vi "Process.vi"(8 "error in":errorcluster) -> (0 "error out":errorcluster)   [LabVIEW 2021, in "dcvmDPI_AD7606B_serverImpl.lvlib"]
uses:
  dcvmDPI_AD7606B_serverImpl.lvlib
  controls/configuration.ctl
  controls/session.ctl
  dcvmDPI_AD7606B_server/RPC Messages/dcvmDPI_IdResponse.ctl
  dcvmDPI_AD7606B_server/RPC Messages/dcvmDPI_ErrorResponse.ctl
  dcvmMessageQueue/controls/Message Data.ctl
  dcvmDPI_AD7606B_server/RPC Messages/dcvmDPI_MeasurementRequest.ctl
  dcvmDPI_AD7606B_server/RPC Messages/dcvmDPI_MeasurementResponse.ctl
  dcvmDPI_AD7606B_server/RPC Messages/dcvmDPI_InitializeRequest.ctl
  dcvmDPI_AD7606B_server/RPC Messages/dcvmDPI_InitializeResponse.ctl
  <instrlib>/niDigital/niDigital.llb/niDigital Trigger Digital Edge - Edge.ctl
  dcvmDPI_AD7606B_server/RPC Messages/dcvmDPI_ConfigureRequest.ctl
  dcvmDPI_AD7606B_server/RPC Messages/dcvmDPI_ConfigureResponse.ctl
  dcvmDPI_AD7606B_server/RPC Messages/dcvmDPI_InitiateResponse.ctl
  dcvmDPI_AD7606B_server/RPC Messages/dcvmDPI_CloseResponse.ctl
  dcvmMessageQueue/dcvmMessageQueue.lvlib
  dcvmDPI_AD7606B_server/dcvmDPI_AD7606B_server.lvlib
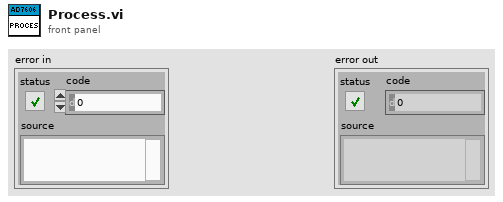
[diagram p1: front panel]
types:
  T1 = typedef "dcvmDPI_AD7606B_serverImpl.lvlib/session.ctl" = cluster{"DPI session":refnum<k15>, "DPI bitfile reference":refnum<k20>}
  T2 = typedef "dcvmDPI_AD7606B_serverImpl.lvlib/configuration.ctl" = cluster{"Input channel":i32, "Sample rate":dbl, "Number of samples":u32, "Measurement Name":string, "reg 0":i32, "reg 1":i32, "Delay ?":bool}
  T3 = typedef "dcvmMessageQueue.lvlib/Message Queues.ctl" = cluster{"gRPC engine":refnum<queue>, "Digital engine":refnum<queue>}
  T4 = typedef "dcvmMessageQueue.lvlib/Message Data.ctl" = cluster{"Action":string, "Value":variant}
  T5 = typedef "dcvmDPI_AD7606B_server.lvlib/dcvmDPI_IdResponse.ctl" = cluster{"name":string, "error":T6}
  T6 = typedef "dcvmDPI_AD7606B_server.lvlib/dcvmDPI_ErrorResponse.ctl" = cluster{"error_number":i32, "error_description":string}
  T7 = typedef "dcvmDPI_AD7606B_server.lvlib/dcvmDPI_MeasurementResponse.ctl" = cluster{"error":T6}
  T8 = typedef "dcvmDPI_AD7606B_server.lvlib/dcvmDPI_MeasurementRequest.ctl" = cluster{"measurement":string}
  T9 = typedef "dcvmDPI_AD7606B_server.lvlib/dcvmDPI_InitializeResponse.ctl" = cluster{"error":T6}
  T10 = typedef "dcvmDPI_AD7606B_server.lvlib/dcvmDPI_InitializeRequest.ctl" = cluster{"device_name":string}
  T11 = typedef "dcvmDPI_AD7606B_server.lvlib/dcvmDPI_ConfigureResponse.ctl" = cluster{"error":T6}
  T12 = enum16{"Initialize", "Write", "Read", "GetBacklog", "Reset"}
  T13 = typedef "dcvmDPI_AD7606B_server.lvlib/dcvmDPI_ConfigureRequest.ctl" = cluster{"digital_capture_samples":u32, "digital_capture_sample_rate":dbl, "input_channel":i32}
  T14 = typedef "dcvmDPI_AD7606B_server.lvlib/dcvmDPI_InitiateResponse.ctl" = cluster{"error":T6}
  T15 = typedef "dcvmDPI_AD7606B_server.lvlib/dcvmDPI_CloseResponse.ctl" = cluster{"error":T6}
  T16 = typedef "niDigital Trigger Digital Edge - Edge.ctl" = i32
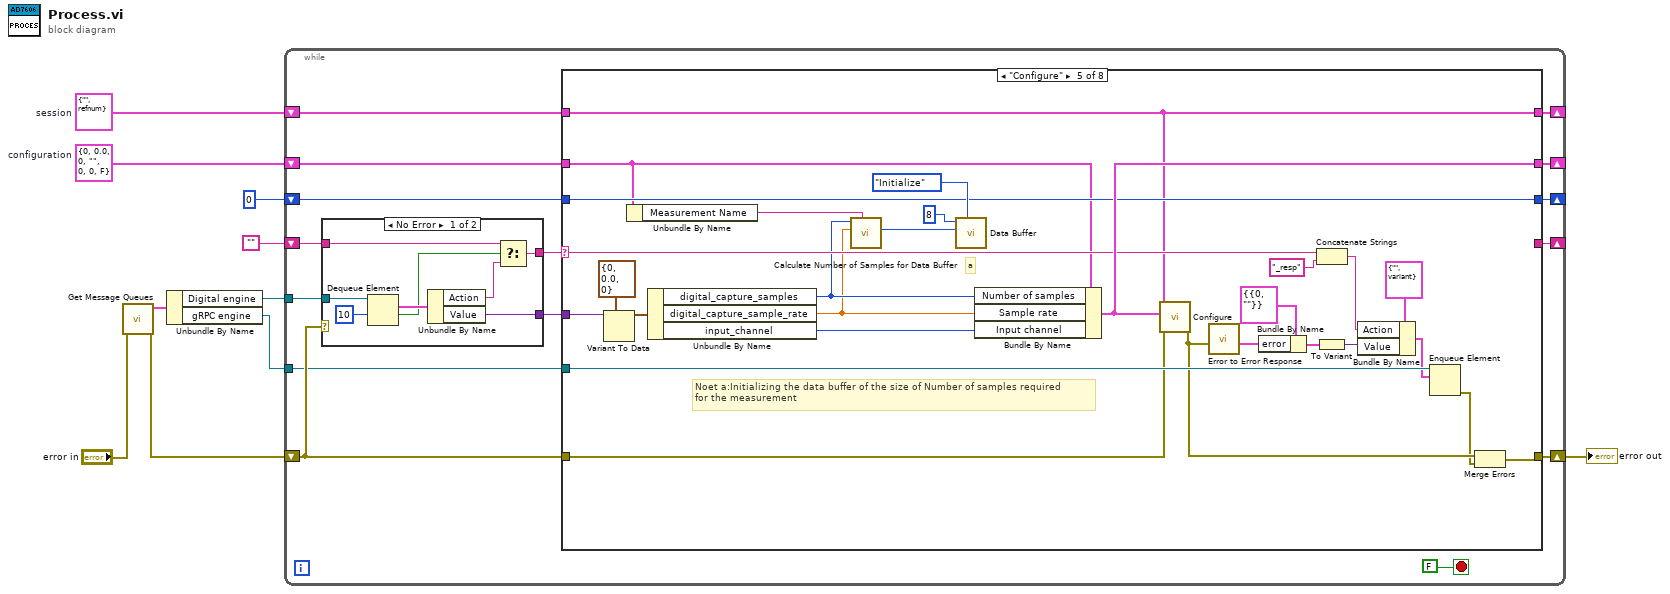
[diagram p0: block diagram]
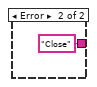
[diagram p2: hidden frame]
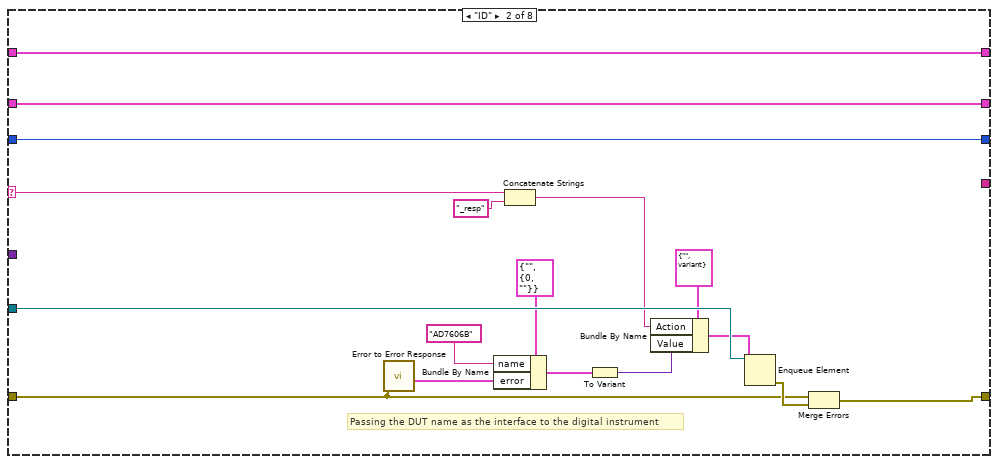
[diagram p4: hidden frame]
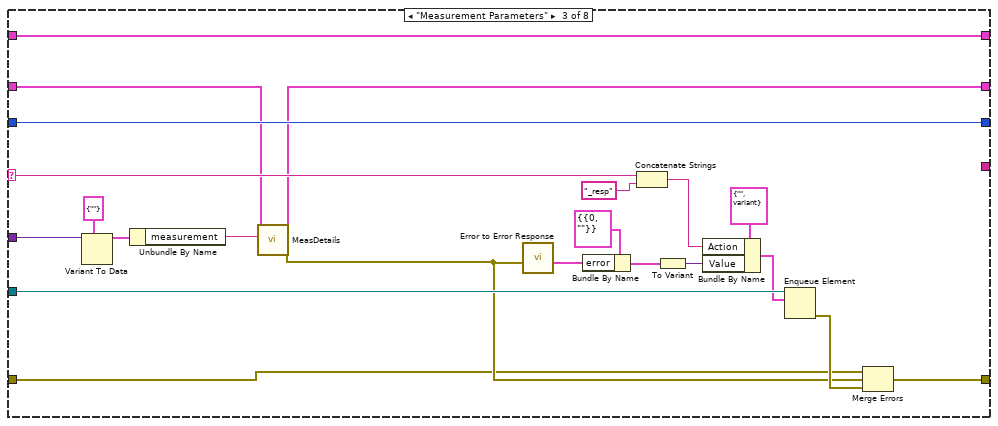
[diagram p5: hidden frame]
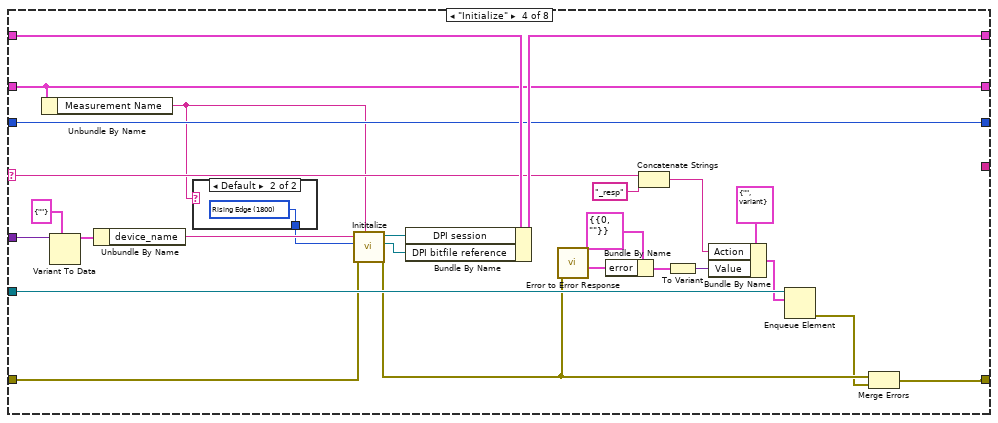
[diagram p6: hidden frame]
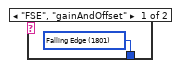
[diagram p7: hidden frame]
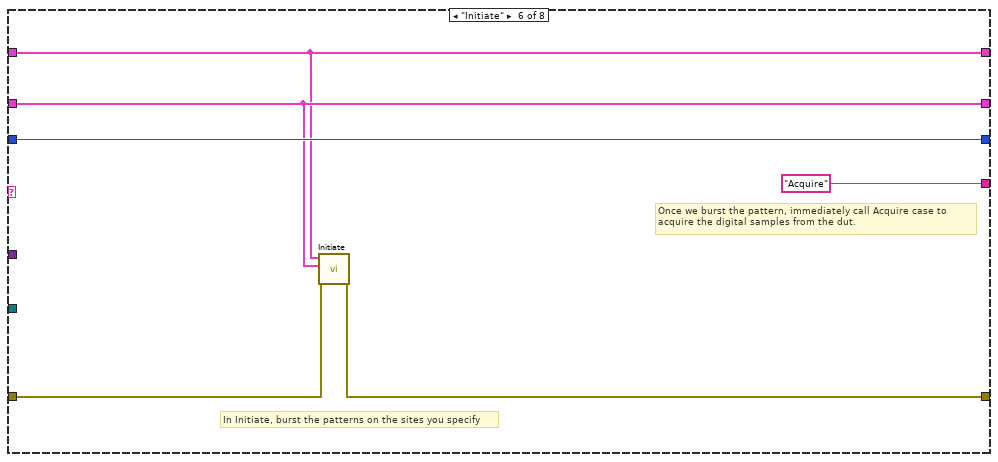
[diagram p8: hidden frame]
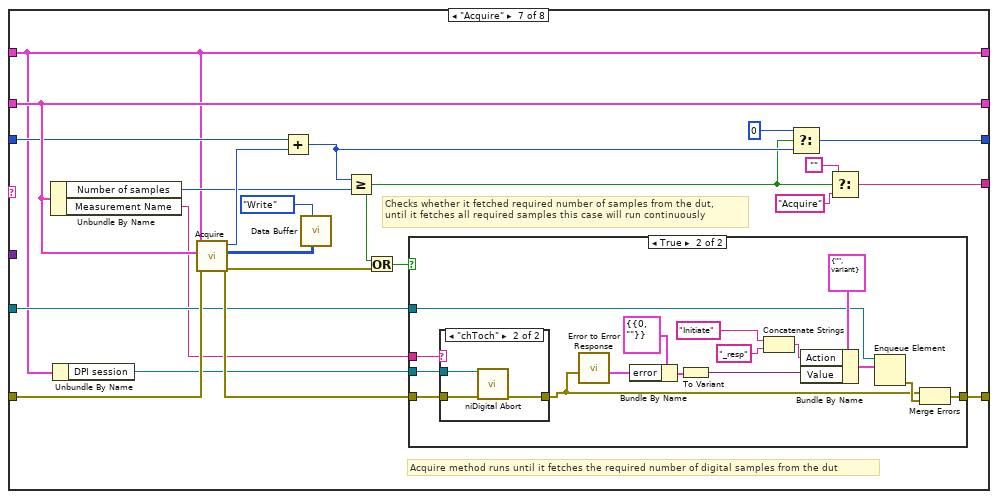
[diagram p9: hidden frame]
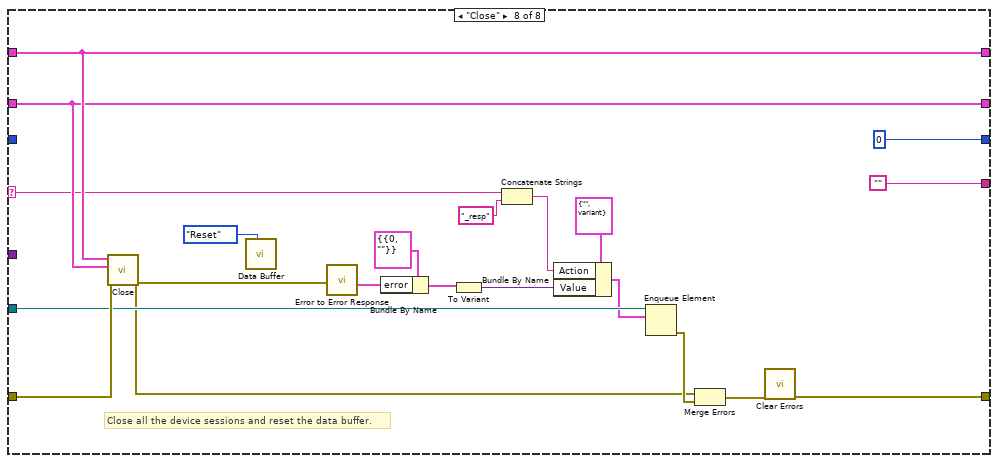
[diagram p12: hidden frame]
diagram:
  w10 = T1 {"DPI session"="", "DPI bitfile reference"=refnum}  # session
  w9 = T2 {"Input channel"=0, "Sample rate"=0.0, "Number of samples"=0, "Measurement Name"="", "reg 0"=0, "reg 1"=0, "Delay ?"=FALSE}  # configuration
  n1 = call "Get Message Queues.vi"("error in (no error)"="error in") -> ("error out"=w3:errorcluster, "AllMsgQueues QueueRef"=w7:T3)  [unwired: 8 in, 1 out]
  n2 = Unbundle By Name(w7) -> ("Digital engine"=w6:refnum<queue>, "gRPC engine"=w4:refnum<queue>)
  n3 = while {
    shift-right: [w16] -> _
    shift-left: w10 -> [w17]
    shift-right: [w18] -> _
    shift-left: w9 -> [w19]
    tunnel: w6 -> [w25]
    tunnel: w4 -> [w11]
    shift-right: [w20] -> w2
    shift-left: w3 -> [w12]
    shift-right: [w15] -> _
    shift-left: "" -> [w23]
    shift-right: [w13] -> _
    shift-left: u32 0 -> [w14]
    stop <- FALSE stop-if-true
    n4 = case shown="No Error" w12 {
      tunnel: w25 -> [w33 _]
      tunnel: [w31 _] -> w24
      tunnel: w23 -> [w27 _]
      tunnel: [w26 "Close" ("Action")] -> w22
      frame No Error {
        n5 = Dequeue Element(queue=w33, timeout in ms (-1)=10) -> (element=w32:T4, timed out?=w29:bool)  [unwired: 1 in, 2 out]
        n6 = Unbundle By Name(w32) -> ("Action"=w28:string, "Value"=w31:variant)
        n7 = Select(t=w27, s=w29, f=w28) -> (s? t:f=w26:string)
      }
      frame Error {
      }
    }
    n8 = case shown="\"Configure\"" w22 {
      selector: w22 -> [_ w48 w75 w93 w128 _ _ w197]
      tunnel: w24 -> [_ _ w70 w103 w133 _ _ _]
      tunnel: w11 -> [_ w51 w77 w94 w129 _ w150 w195]
      tunnel: w12 -> [w36 w39 w56 w82 w115 w138 w160 w199]
      tunnel: [w36 w41 w64 w85 w118 w135 w151 w183] -> w20
      tunnel: w19 -> [w37 w52 w59 w88 w107 w137 w158 w200]
      tunnel: [w37 w52 w58 w88 w130 w137 w158 w200] -> w18
      tunnel: w17 -> [w38 w53 w71 w98 w111 w136 w141 w201]
      tunnel: [w38 w53 w71 w95 w111 w136 w141 w201] -> w16
      tunnel: [_ _ _ _ _ "Acquire" w155 ""] -> w15
      tunnel: w14 -> [w35 w49 w67 w87 w121 w139 w157 _]
      tunnel: [w35 w49 w67 w87 w121 w139 w146 u32 0] -> w13
      frame "", Default {
      }
      frame "ID" {
        # "Passing the DUT name as the interface to the digital instrument"
        n9 = call "Error to Error Response.vi"("error in (no error)"=w39) -> ("error response"=w55:T6)  [unwired: 10 in]
        n10 = Bundle By Name(cluster=T5 {"name"="", "error"={"error_number"=0, "error_description"=""}} ("dcvmDigitalInterface_IdResponse"), "name"="AD7606B", "error"=w55) -> (w43:T5)
        n11 = Concatenate Strings(w48, "_resp" ("string")) -> (w45:string)
        n12 = To Variant(anything=w43) -> (Variant=w42:variant)
        n13 = Bundle By Name(cluster=T4 {"Action"="", "Value"=variant} ("Message data"), "Action"=w45, "Value"=w42) -> (w44:T4)
        n14 = Enqueue Element(queue=w51, element=w44) -> (error out=w40:errorcluster)  [unwired: 2 in, 2 out]
        n15 = Merge Errors(w39, w40) -> (w41:errorcluster)
      }
      frame "Measurement Parameters" {
        n16 = Variant To Data(type=T8 {"measurement"=""} ("dcvmDigitalInterface_MeasurementRequest"), Variant=w70) -> (data=w68:T8)  [unwired: 1 in, 1 out]
        n17 = Unbundle By Name(w68) -> ("measurement"=w60:string)
        n18 = call "MeasDetails.vi"("measurement"=w60, "Configuration In"=w59) -> ("error out"=w57:errorcluster, "Configuration out"=w58:T2)  [unwired: 8 in]
        n19 = call "Error to Error Response.vi"("error in (no error)"=w57) -> ("error response"=w65:T6)  [unwired: 10 in]
        n20 = Bundle By Name(cluster=T7 {"error"={"error_number"=0, "error_description"=""}} ("dcvmDigitalInterface_MeasurementResponse"), "error"=w65) -> (w62:T7)
        n21 = Concatenate Strings(w75, "_resp" ("string")) -> (w73:string)
        n22 = To Variant(anything=w62) -> (Variant=w61:variant)
        n23 = Bundle By Name(cluster=T4 {"Action"="", "Value"=variant} ("Message data"), "Action"=w73, "Value"=w61) -> (w72:T4)
        n24 = Enqueue Element(queue=w77, element=w72) -> (error out=w63:errorcluster)  [unwired: 2 in, 2 out]
        n25 = Merge Errors(w56, w57, w63) -> (w64:errorcluster)
      }
      frame "Initialize" {
        n26 = Unbundle By Name(w88) -> ("Measurement Name"=w78:string)
        n27 = Variant To Data(type=T10 {"device_name"=""} ("dcvmDigitalInterface_InitializeRequest"), Variant=w103) -> (data=w101:T10)  [unwired: 1 in, 1 out]
        n28 = Unbundle By Name(w101) -> ("device_name"=w100:string)
        n29 = case shown="Default" w78 {
          tunnel: [w104 w105] -> w99
          frame "FSE", "gainAndOffset" {
            w104 = T16 1801 items=["Rising Edge"=1800, "Falling Edge"=1801] ("TriggerEdge")
          }
          frame Default {
            w105 = T16 1800 items=["Rising Edge"=1800, "Falling Edge"=1801] ("TriggerEdge")
          }
        }
        n30 = call "Inititalize.vi"("Active measurement"=w78, "error in"=w82, "Trigger edge"=w99, "DPI resource name"=w100) -> ("error out"=w84:errorcluster, "DPI Bitfile reference"=w96:refnum<k20>, "DPI Session"=w97:refnum<k15>)  [unwired: 5 in]
        n31 = Bundle By Name(cluster=w98, "DPI session"=w97, "DPI bitfile reference"=w96) -> (w95:T1)
        n32 = call "Error to Error Response.vi"("error in (no error)"=w84) -> ("error response"=w79:T6)  [unwired: 10 in]
        n33 = Bundle By Name(cluster=T9 {"error"={"error_number"=0, "error_description"=""}} ("dcvmDPI_InitializeResponse"), "error"=w79) -> (w81:T9)
        n34 = Concatenate Strings(w93, "_resp" ("string")) -> (w90:string)
        n35 = To Variant(anything=w81) -> (Variant=w86:variant)
        n36 = Bundle By Name(cluster=T4 {"Action"="", "Value"=variant} ("Message data"), "Action"=w90, "Value"=w86) -> (w89:T4)
        n37 = Enqueue Element(queue=w94, element=w89) -> (error out=w83:errorcluster)  [unwired: 2 in, 2 out]
        n38 = Merge Errors(w84, w83) -> (w85:errorcluster)
      }
      frame "Configure" {
        # "a"
        # "Noet a:Initializing the data buffer of the size of Number of samples required\nfor the measurement"
        n39 = Variant To Data(type=T13 {"digital_capture_samples"=0, "digital_capture_sample_rate"=0.0, "input_channel"=0} ("dcvmDigitalInterface_ConfigureRequest"), Variant=w133) -> (data=w131:T13)  [unwired: 1 in, 1 out]
        n40 = Unbundle By Name(w107) -> ("Measurement Name"=w106:string)
        n41 = Unbundle By Name(w131) -> ("digital_capture_samples"=w109:u32, "digital_capture_sample_rate"=w108:dbl, "input_channel"=w122:i32)
        n42 = call "Calculate Number of Samples for Data Buffer.vi"("Measurement"=w106, "Sample rate"=w108, "Number of samples"=w109) -> ("Total no of samples per channel"=w110:u32)  [unwired: 8 in]
        n43 = call "Data Buffer.vi"("Operation"=T12."Initialize", "Samples per channel"=w110, "Channels"=8) -> ()  [unwired: 7 in, 2 out]
        n44 = Bundle By Name(cluster=w107, "Number of samples"=w109, "Sample rate"=w108, "Input channel"=w122) -> (w130:T2)
        n45 = call "Configure.vi"("error in"=w115, "configuration"=w130, "session in"=w111) -> ("error out"=w117:errorcluster)  [unwired: 8 in]
        n46 = call "Error to Error Response.vi"("error in (no error)"=w117) -> ("error response"=w113:T6)  [unwired: 10 in]
        n47 = Bundle By Name(cluster=T11 {"error"={"error_number"=0, "error_description"=""}} ("dcvmDPI_ConfigureResponse"), "error"=w113) -> (w112:T11)
        n48 = Concatenate Strings(w128, "_resp" ("string")) -> (w124:string)
        n49 = To Variant(anything=w112) -> (Variant=w119:variant)
        n50 = Bundle By Name(cluster=T4 {"Action"="", "Value"=variant} ("Message data"), "Action"=w124, "Value"=w119) -> (w126:T4)
        n51 = Enqueue Element(queue=w129, element=w126) -> (error out=w116:errorcluster)  [unwired: 2 in, 2 out]
        n52 = Merge Errors(w117, w116) -> (w118:errorcluster)
      }
      frame "Initiate" {
        # "Once we burst the pattern, immediately call Acquire case to \nacquire the digital samples from the dut."
        # "In Initiate, burst the patterns on the sites you specify"
        n53 = call "Initiate.vi"("error in"=w138, "configuration"=w137, "session in"=w136) -> ("error out"=w135:errorcluster)  [unwired: 8 in]
      }
      frame "Acquire" {
        # "Checks whether it fetched required number of samples from the dut,\nuntil it fetches all required samples this case will run continuously"
        # "Acquire method runs until it fetches the required number of digital samples from the dut"
        n54 = Unbundle By Name(w158) -> ("Number of samples"=w148:u32, "Measurement Name"=w142:string)
        n55 = Unbundle By Name(w141) -> ("DPI session"=w140:refnum<k15>)
        n56 = call "Acquire.vi"("error in"=w160, "configuration"=w158, "session"=w141) -> ("error out"=w152:errorcluster, "Digital waveform"=w154:u32[][], "No of Samples per channel"=w149:u32)  [unwired: 6 in]
        n57 = Add(x=w157, y=w149) -> (x+y=w145:u32)
        n58 = call "Data Buffer.vi"("Data in"=w154, "Operation"=T12."Write") -> ()  [unwired: 8 in, 2 out]
        n59 = Greater Or Equal?(x=w145, y=w148) -> (x >= y?=w143:bool)
        n60 = Or(x=w143, y=w152) -> (x .or. y?=w153:bool)
        n61 = case shown="True" w153 {
          tunnel: w152 -> [w161 w165]
          tunnel: [w161 w169] -> w151
          tunnel: w150 -> [_ w166]
          tunnel: w142 -> [_ w163]
          tunnel: w140 -> [_ w162]
          frame False {
          }
          frame True {
            n62 = case shown="\"chToch\"" w163 {
              tunnel: w165 -> [w178 w181]
              tunnel: [w178 w180] -> w164
              tunnel: w162 -> [_ w179]
              frame Default {
              }
              frame "chToch" {
                n63 = call <instrlib>:"niDigital Abort.vi"("instrument handle"=w179, "error in"=w181) -> ("error out"=w180:errorcluster)  [unwired: 12 in, 1 out]
              }
            }
            n64 = call "Error to Error Response.vi"("error in (no error)"=w164) -> ("error response"=w170:T6)  [unwired: 10 in]
            n65 = Bundle By Name(cluster=T14 {"error"={"error_number"=0, "error_description"=""}} ("dcvmDPI_InitiateResponse"), "error"=w170) -> (w172:T14)
            n66 = To Variant(anything=w172) -> (Variant=w175:variant)
            n67 = Concatenate Strings("Initiate" ("string"), "_resp" ("string")) -> (w174:string)
            n68 = Bundle By Name(cluster=T4 {"Action"="", "Value"=variant} ("Message data"), "Action"=w174, "Value"=w175) -> (w176:T4)
            n69 = Enqueue Element(queue=w166, element=w176) -> (error out=w168:errorcluster)  [unwired: 2 in, 2 out]
            n70 = Merge Errors(w164, w168) -> (w169:errorcluster)
          }
        }
        n71 = Select(t=u32 0, s=w143, f=w145) -> (s? t:f=w146:u32)
        n72 = Select(t="", s=w143, f="Acquire") -> (s? t:f=w155:string)
      }
      frame "Close" {
        # "Close all the device sessions and reset the data buffer."
        n73 = call "Close.vi"("error in"=w199, "configuration"=w200, "session"=w201) -> ("error out"=w186:errorcluster)  [unwired: 8 in]
        n74 = call "Data Buffer.vi"("Operation"=T12."Reset") -> ()  [unwired: 9 in, 2 out]
        n75 = call "Error to Error Response.vi"("error in (no error)"=w186) -> ("error response"=w193:T6)  [unwired: 10 in]
        n76 = Bundle By Name(cluster=T15 {"error"={"error_number"=0, "error_description"=""}} ("dcvmDigitalInterface_CloseResponse"), "error"=w193) -> (w191:T15)
        n77 = To Variant(anything=w191) -> (Variant=w190:variant)
        n78 = Concatenate Strings(w197, "_resp" ("string")) -> (w189:string)
        n79 = Bundle By Name(cluster=T4 {"Action"="", "Value"=variant} ("Message data"), "Action"=w189, "Value"=w190) -> (w188:T4)
        n80 = Enqueue Element(queue=w195, element=w188) -> (error out=w187:errorcluster)  [unwired: 2 in, 2 out]
        n81 = Merge Errors(w186, w187) -> (w184:errorcluster)
        n82 = call <vilib>:"Clear Errors.vi"("error in (no error)"=w184) -> ("error out"=w183:errorcluster)  [unwired: 5 in, 1 out]
      }
    }
  }
  "error out" <- w2
